vi "CircularRadius.vi"(0 "controller in":refnum<k24>, 1 "axis 1 name":string, 2 "axis 1 endpoint":dbl, 3 "axis 2 name":string, 4 "axis 2 endpoint":dbl, 5 "error in (no error)":errorcluster, 6 "speed":dbl, 7 "radius":dbl, 8 "direction":u16(ring) items=["Clockwise", "Counter-clockwise"], 9 "return immediately":bool) -> (14 "controller out":refnum<k24>, 19 "error out":errorcluster)   [LabVIEW 2010]
uses:
  c:/aerotech/controller/5.xx.xxx/ensemble/pc/labview/2010/bin/Aerotech.Ensemble.dll
  bin/Aerotech.Ensemble.dll
  c:/aerotech/controller/5.xx.xxx/ensemble/pc/labview/2010/bin/Aerotech.Ensemble.LabVIEW.dll
  bin/Aerotech.Ensemble.LabVIEW.dll
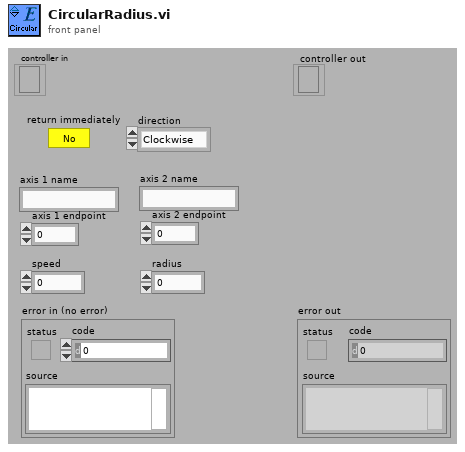
[diagram p1: front panel]
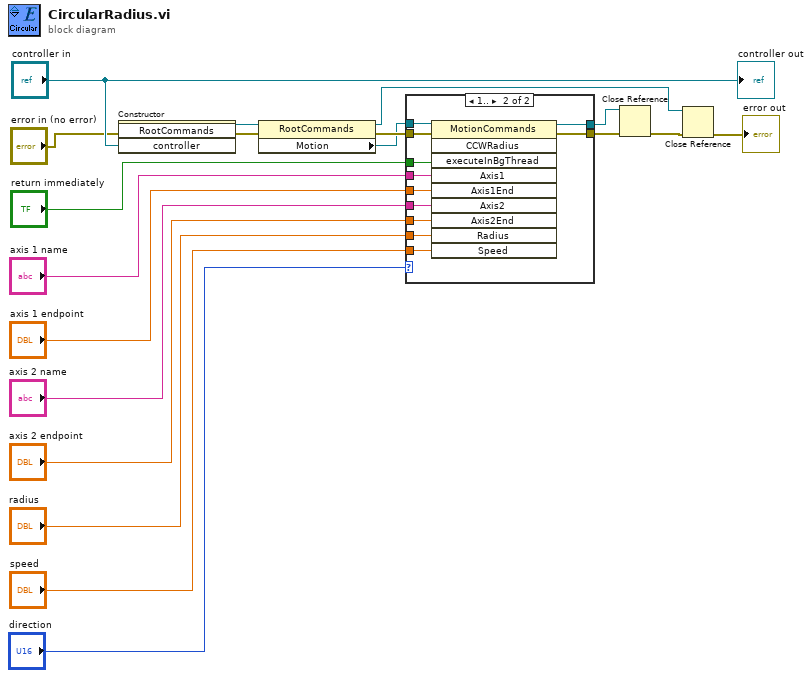
[diagram p0: block diagram]
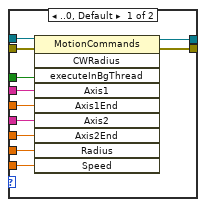
[diagram p2: hidden frame]
diagram:
  n1 = constructor class="RootCommands"(error in="error in (no error)", "controller"="controller in") -> (reference out=w3:refnum<k24>, error out=w4:errorcluster)  [unwired: 2 in, 2 out]
  n2 = property class="RootCommands"(reference=w3, error in=w4) -> (reference out=w8:refnum<k24>, error out=w2:errorcluster, "Motion"=w1:refnum<k24>)
  n3 = case shown="1.." "direction" {
    tunnel: [w30 w39] -> w6
    tunnel: [w29 w38] -> w5
    tunnel: w2 -> [w28 w41]
    tunnel: w1 -> [w27 w40]
    tunnel: "speed" -> [w26 w37]
    tunnel: "radius" -> [w25 w36]
    tunnel: "axis 2 endpoint" -> [w24 w35]
    tunnel: "axis 1 name" -> [w23 w32]
    tunnel: "axis 1 endpoint" -> [w22 w33]
    tunnel: "axis 2 name" -> [w21 w34]
    tunnel: "return immediately" -> [w20 w31]
    frame ..0, Default {
      n4 = invoke class="MotionCommands" method="CWRadius"(reference=w27, error in=w28, "executeInBgThread"=w20, "Axis1"=w23, "Axis1End"=w22, "Axis2"=w21, "Axis2End"=w24, "Radius"=w25, "Speed"=w26) -> (reference out=w30:refnum<k24>, error out=w29:errorcluster)  [unwired: 1 in, 8 out]
    }
    frame 1.. {
      n5 = invoke class="MotionCommands" method="CCWRadius"(reference=w40, error in=w41, "executeInBgThread"=w31, "Axis1"=w32, "Axis1End"=w33, "Axis2"=w34, "Axis2End"=w35, "Radius"=w36, "Speed"=w37) -> (reference out=w39:refnum<k24>, error out=w38:errorcluster)  [unwired: 1 in, 8 out]
    }
  }
  n6 = Close Reference(reference=w6, error in (no error)=w5) -> (error out=w7:errorcluster)
  n7 = Close Reference(reference=w8, error in (no error)=w7) -> (error out=→"error out":errorcluster)
  "controller out" <- "controller in"
